vi "Load Profile.vi"(0 "Output":bool, 5 "References":refnum<vi>[](array[refnum])) -> (4 "error out":errorcluster)   [LabVIEW 2016]
uses:
  <vilib>/Utility/file.llb/Read Delimited Spreadsheet (DBL).vi
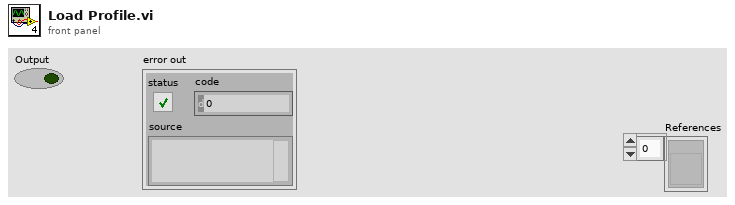
[diagram p1: front panel]
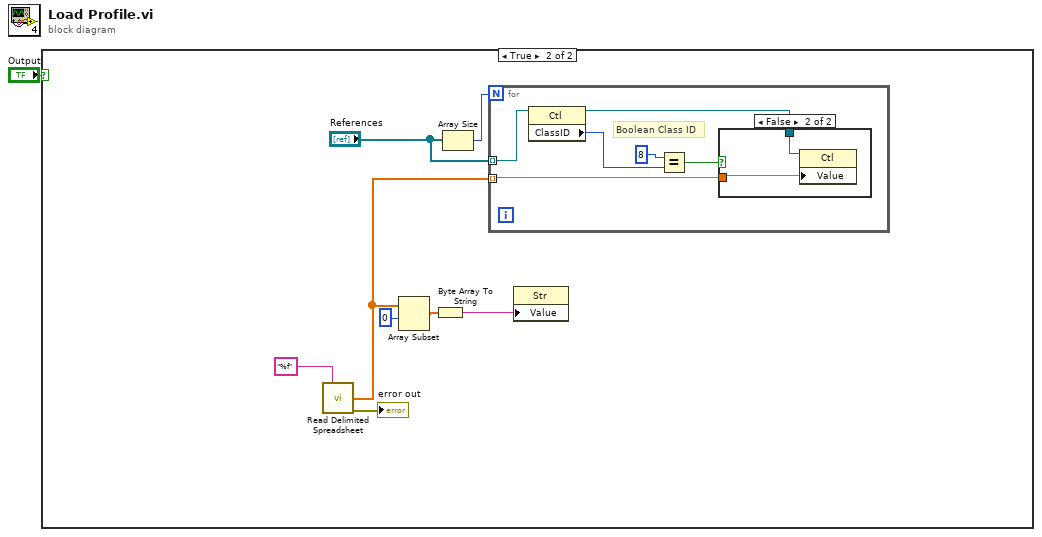
[diagram p0: block diagram]
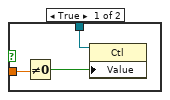
[diagram p3: hidden frame]
diagram:
  n1 = case shown="True" "Output" {
    frame False {
    }
    frame True {
      n2 = call-poly <vilib>:"Read Delimited Spreadsheet.vi"("format (%.3f)"="%f") -> ("first row"=w5:dbl[], "error out"=→"error out":errorcluster)  [unwired: 9 in, 4 out]
      n3 = Array Subset(array=w5, index=0) -> (w2:dbl[])  [unwired: 1 in]
      n4 = Byte Array To String(unsigned byte array=w2) -> (string=w7:string)
      n5 = Array Size(array="References") -> (size(s)=w4:i32)
      n6 = for {
        N: w4 -> [_]
        tunnel: w5 -> [w11] mode=indexing
        tunnel: "References" -> [w15] mode=indexing
        # "Boolean Class ID"
        n7 = property class="Ctl"(reference=w15) -> (reference out=w10:refnum<vi>, "ClassID"=w14:u32)  [unwired: 1 in, 1 out]
        n8 = Equal?(x=u32 8, y=w14) -> (x = y?=w12:bool)
        n9 = case shown="False" w12 {
          tunnel: w11 -> [w18 w19]
          tunnel: w10 -> [w16 w20]
          frame True {
            n10 = Not Equal To 0?(x=w18) -> (x != 0?=w17:bool)
            n11 = property class="Ctl"(reference=w16, "Value"=w17) -> ()  [unwired: 1 in, 2 out]
          }
          frame False {
            n12 = property class="Ctl"(reference=w20, "Value"=w19) -> ()  [unwired: 1 in, 2 out]
          }
        }
      }
      n13 = property on="Property Node" class="Str"("Value"=w7) -> ()  [unwired: 2 in, 2 out]
    }
  }
